vi "ZAlign_CtrlsAvail.vi"(10 "ConectedRefs":refnum<vi>[](array[refnum]), 11 "LocalRefs":refnum<vi>[](array[refnum])) -> (2 "ConRefsAvail":bool, 3 "RefsAvail":bool)   [LabVIEW 2014, in "ZAlign.lvlib"]
doc: "ZAlign.lvlib:ZAlign_CtrlsAvail.vi\n----------------------------------------------\nControls gefunden/selektiert?\n\nInputs:\n---------------------\n- ConectedRefs : 1DArrayOfRefnum; \n- LocalRefs : 1DArrayOfRefnum; \n\nOutputs:\n---------------------\n- ConRefsAvail : Boolean; \n- RefsAvail : Boolean; \n\n----------------------------------------------\n26.03.2015 jcm\nZühlke Engineering AG\nCH-8952 Schlieren\nwww.zuehlke.com"
uses:
  ZAlign.lvlib
panel:
  # "Connector Pane"
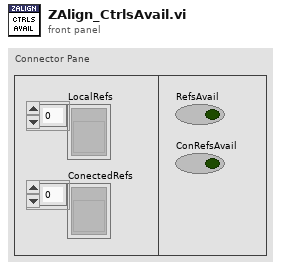
[diagram p1: front panel]
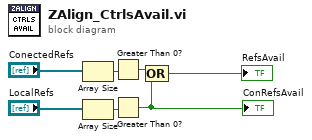
[diagram p0: block diagram]
diagram:
  n1 = Array Size(array="ConectedRefs") -> (size(s)=w3:i32)
  n2 = Array Size(array="LocalRefs") -> (size(s)=w2:i32)
  n3 = Greater Than 0?(x=w3) -> (x > 0?=w5:bool)
  n4 = Greater Than 0?(x=w2) -> (x > 0?=w6:bool)
  "ConRefsAvail" <- w6
  n5 = Compound Arithmetic op=OR(w5, w6) -> (→"RefsAvail":bool)
